vi "PBKDF2 Main.vi"(1 "SSID":u8[](array[numeric]), 2 "Secret Key":u8[](array[numeric])) -> (0 "PSK":u8[](array[numeric]))   [LabVIEW 2014]
panel:
  # "Secret Key is the password entered into the router or our current guess\n\nSalt is the SSID."
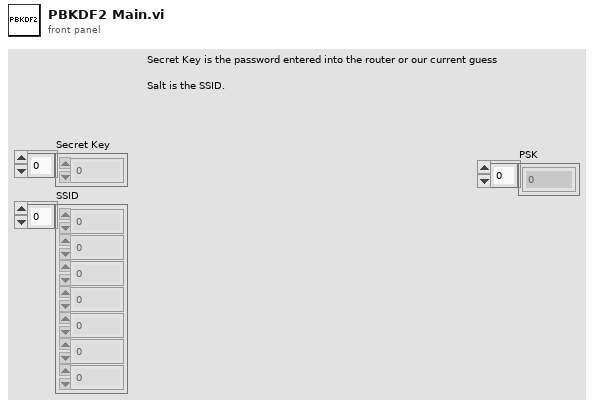
[diagram p1: front panel]
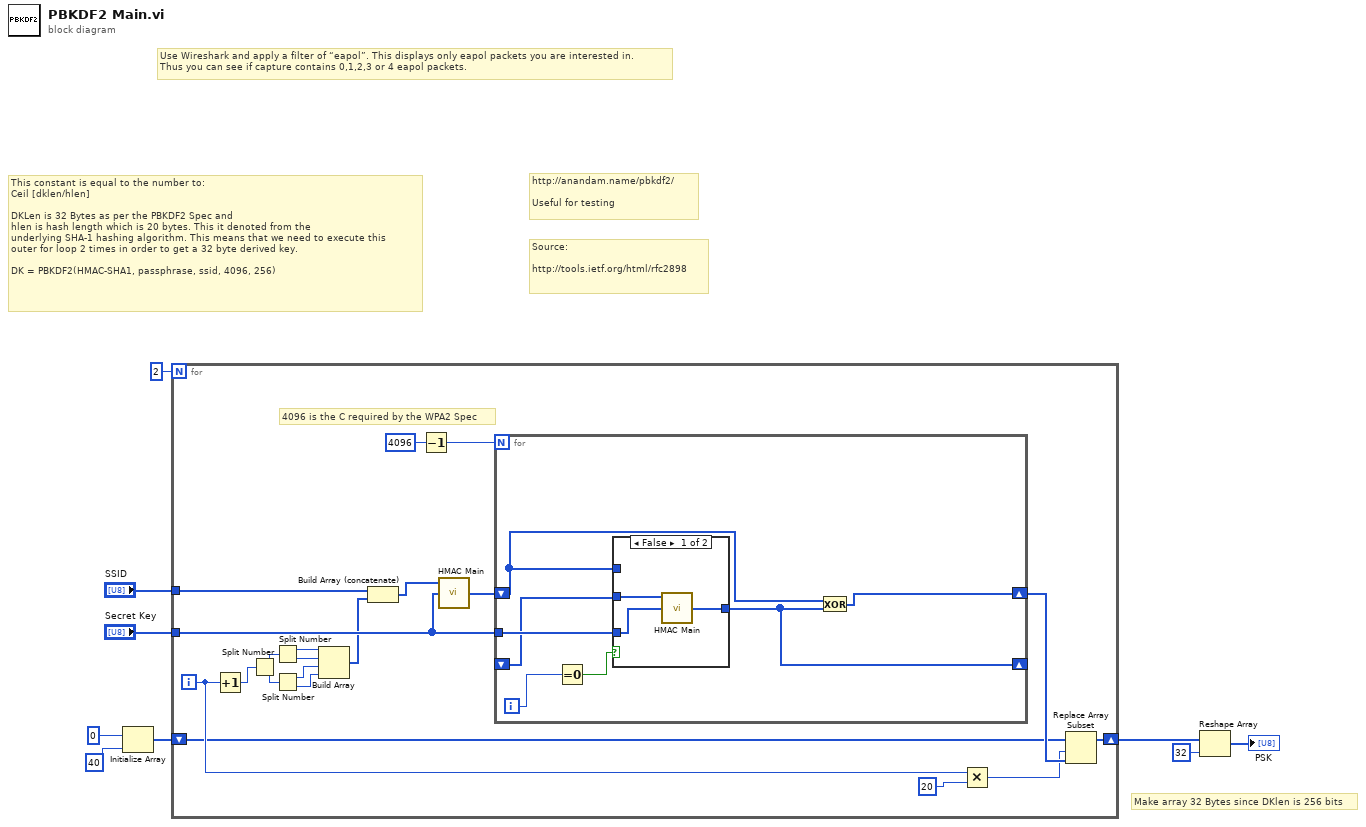
[diagram p0: block diagram]
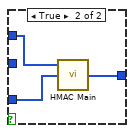
[diagram p2: hidden frame]
diagram:
  # "Make array 32 Bytes since DKlen is 256 bits"
  # "Use Wireshark and apply a filter of “eapol”. This displays only eapol packets you are interested in. \nThus you can see if capture contains 0,1,2,3 or 4 eapol packets."
  # "http://anandam.name/pbkdf2/\n\nUseful for testing"
  # "This constant is equal to the number to:\nCeil [dklen/hlen]\n\nDKLen is 32 Bytes as per the PBKDF2 Spec and \nhlen is hash length which is 20 bytes. This it denoted from the \nunderlying SHA-1 hashing algorithm. This means that we need to execute this\nouter for loop 2 times in order to get a 32 byte derived key.\n\nDK = PBKDF2(HMAC-SHA1, passphrase, ssid, 4096, 256)"
  # "Source:\n\nhttp://tools.ietf.org/html/rfc2898"
  n1 = Initialize Array(u8 0, 40 ("dimension size")) -> (w1:u8[])
  n2 = for {
    N: 2 -> [_]
    tunnel: "Secret Key" -> [w26]
    tunnel: "SSID" -> [w29]
    shift-right: [w10] -> w8
    shift-left: w1 -> [w11]
    i -> [w14]
    # "4096 is the C required by the WPA2 Spec"
    n3 = Increment(x=w14) -> (x+1=w20:i32)
    n4 = Split Number(x=w20) -> (hi(x)=w21:u16, lo(x)=w19:u16)
    n5 = Split Number(x=w21) -> (hi(x)=w25:u8, lo(x)=w24:u8)
    n6 = Split Number(x=w19) -> (hi(x)=w23:u8, lo(x)=w22:u8)
    n7 = Build Array(w25, w24, w23, w22) -> (w18:u8[])
    n8 = Build Array (concatenate)(w29, w18) -> (w28:u8[])
    n9 = Decrement(x=4096) -> (x-1=w17:i32)
    n10 = call "HMAC Main.vi"("Secret Key"=w26, "Message"=w28) -> ("HMAC Out"=w27:u8[])  [unwired: 1 in]
    n11 = for {
      N: w17 -> [_]
      tunnel: w26 -> [w36]
      shift-right: [w34] -> _
      shift-left: _ -> [w33]
      shift-right: [w35] -> w15
      shift-left: w27 -> [w30]
      i -> [w32]
      n12 = Equal To 0?(x=w32) -> (x = 0?=w31:bool)
      n13 = case shown="False" w31 {
        tunnel: w36 -> [w38 w42]
        tunnel: [w37 w41] -> w34
        tunnel: w33 -> [w39 _]
        tunnel: w30 -> [_ w40]
        frame False {
          n14 = call "HMAC Main.vi"("Secret Key"=w38, "Message"=w39) -> ("HMAC Out"=w37:u8[])  [unwired: 1 in]
        }
        frame True {
          n15 = call "HMAC Main.vi"("Secret Key"=w42, "Message"=w40) -> ("HMAC Out"=w41:u8[])  [unwired: 1 in]
        }
      }
      n16 = Exclusive Or(1:w34, 2:w30) -> (0:w35:u8[])
    }
    n17 = Multiply(x=w14, y=20 ("dimension size")) -> (x*y=w12:i32)
    n18 = Replace Array Subset(array=w11, new element=w15, index=w12) -> (w10:u8[])
  }
  n19 = Reshape Array(w8, 32 ("dimension size")) -> (→"PSK":u8[])
